vi "testserverstream.vi"() -> ()   [LabVIEW 2016]
uses:
  tls classes/connection creator/server acceptor/server acceptor.lvclass
  C:/Users/IEUser/Desktop/libasynclvtls/tls classes/connection creator/connection creator.lvclass
  tls classes/engine context/engine context.lvclass
  tls classes/connection/connection.lvclass
  tls classes/connection creator/connection creator.lvclass
panel:
  out "error out 2":errorcluster
  out "error out":errorcluster
  out "output cluster":cluster{"error code":i32, "data":string}
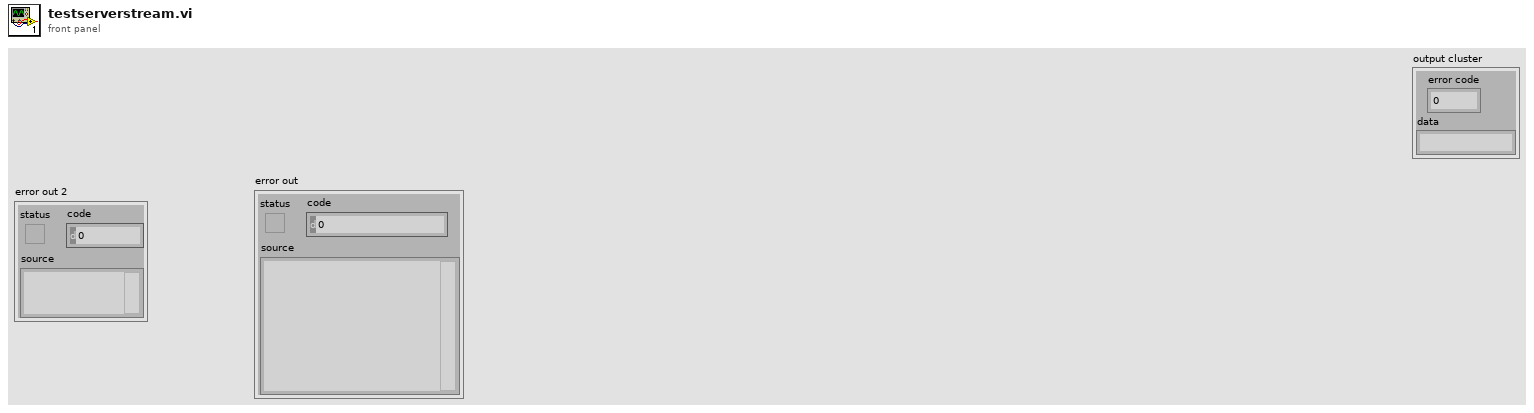
[diagram p1: front panel]
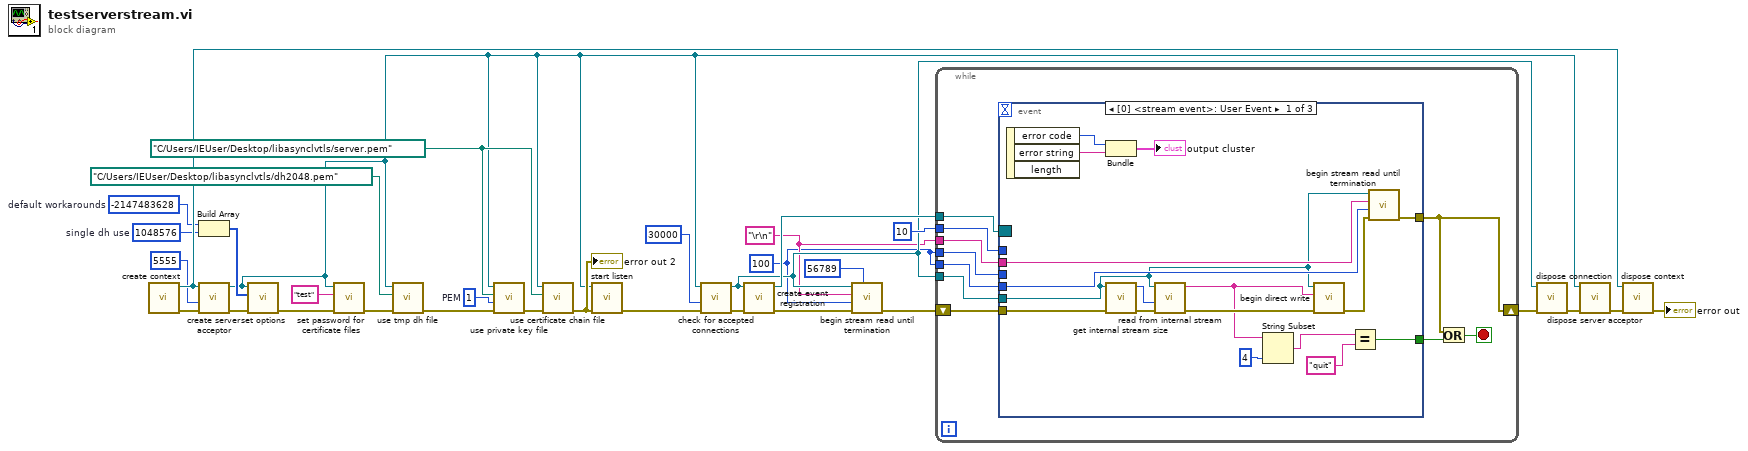
[diagram p0: block diagram]
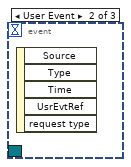
[diagram p2: hidden frame]
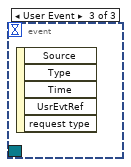
[diagram p3: hidden frame]
diagram:
  w4 = 1  # PEM
  w7 = "\r\n" ("termination")
  w17 = path "C:/Users/IEUser/Desktop/libasynclvtls/server.pem" ("cert chain file")
  w20 = -2147483628  # default workarounds
  w21 = 1048576  # single dh use
  w6 = 100 ("bytes to read")
  n1 = call "create context.vi"() -> ("error out"=w24:errorcluster, "engine context out"=w23:refnum<class "engine context.lvclass">)  [unwired: 10 in]
  n2 = Build Array(w20, w21) -> (w9:i32[])
  n3 = call "create server acceptor.vi"("error in"=w24, "port"=u16 5555, "engine context in"=w23) -> ("error out"=w22:errorcluster, "server acceptor out"=w8:refnum<class "server acceptor.lvclass">)  [unwired: 7 in]
  n4 = call "set options.vi"("error in"=w22, "options"=w9, "connection creator in"=w8) -> ("error out"=w19:errorcluster)  [unwired: 8 in]
  n5 = call "set password for certificate files.vi"("error in"=w19, "password"="test" ("file"), "connection creator in"=w8) -> ("error out"=w3:errorcluster)  [unwired: 8 in]
  n6 = call "use tmp dh file.vi"("error in"=w3, "tmp dh file"=path "C:/Users/IEUser/Desktop/libasynclvtls/dh2048.pem", "connection creator in"=w8) -> ("error out"=w2:errorcluster)  [unwired: 8 in]
  n7 = call "use private key file.vi"("error in"=w2, "format"=w4, "private key file"=w17, "connection creator in"=w8) -> ("error out"=w1:errorcluster)  [unwired: 7 in]
  n8 = call "use certificate chain file.vi"("error in"=w1, "cert chain file"=w17, "connection creator in"=w8) -> ("error out"=w16:errorcluster)  [unwired: 8 in]
  "error out 2" <- w16
  n9 = call "start listen.vi"("error in"=w16, "server acceptor in"=w8) -> ("error out"=w15:errorcluster)  [unwired: 9 in]
  n10 = call "check for accepted connections.vi"("error in"=w15, "timeout"=30000, "server acceptor in"=w8) -> ("error out"=w14:errorcluster, "connection"=w11:refnum<class "connection.lvclass">)  [unwired: 7 in]
  n11 = call "create event registration.vi"("error in"=w14, "connection in"=w11) -> ("error out"=w31:errorcluster, "Event Registration Refnum"=w32:refnum<event-registration>)  [unwired: 8 in]
  n12 = call "begin stream read until termination.vi"("id"=u32 56789, "error in"=w31, "max bytes to read"=w6, "termination"=w7, "connection in"=w11) -> ("error out"=w29:errorcluster)  [unwired: 6 in]
  n13 = while {
    tunnel: w32 -> [w42]
    shift-right: [w36] -> w26
    shift-left: w29 -> [w41]
    tunnel: w11 -> [w40]
    tunnel: 10 ("bytes to read") -> [w39]
    tunnel: w6 -> [w38]
    tunnel: w7 -> [w34]
    tunnel: w6 -> [w33]
    stop <- w37 stop-if-true
    n14 = event shown="[0] <stream event>: User Event" {
      selector: w42 -> [_ _ _]
      dyn-events: _ -> [_ _ _]
      timeout: _ -> [_ _ _]
      tunnel: w41 -> [w46 _ _]
      tunnel: w40 -> [w47 _ _]
      tunnel: [w53 _ _] -> w36
      tunnel: w39 -> [_ _ _]
      tunnel: w38 -> [_ _ _]
      tunnel: [w56 _ _] -> w35
      tunnel: w34 -> [w52 _ _]
      tunnel: w33 -> [w51 _ _]
      event User Event {
        n15 = event-data() -> ("error code"=w59:i32, "error string"=w55:string)  [unwired: 1 in, 1 out]
        n16 = Bundle("error code"=w59, "error string"=w55) -> (→"output cluster":cluster{"error code":i32, "error string":string})  [unwired: 1 in]
        n17 = call "get internal stream size.vi"("error in"=w46, "connection in"=w47) -> ("error out"=w49:errorcluster, "size"=w50:u64)  [unwired: 8 in]
        n18 = call "read from internal stream.vi"("error in"=w49, "max length"=w50, "connection in"=w47) -> ("error out"=w48:errorcluster, "buffer"=w44:string)  [unwired: 7 in]
        n19 = String Subset(string=w44, length (rest)=4 ("length (rest)")) -> (substring=w43:string)  [unwired: 1 in]
        n20 = call "begin direct write.vi"("error in"=w48, "data"=w44, "connection in"=w47) -> ("error out"=w54:errorcluster)  [unwired: 8 in]
        n21 = Equal?(x=w43, y="quit") -> (x = y?=w56:bool)
        n22 = call "begin stream read until termination.vi"("error in"=w54, "max bytes to read"=w51, "termination"=w52, "connection in"=w47) -> ("error out"=w53:errorcluster)  [unwired: 7 in]
      }
      event User Event {
        n23 = event-data() -> ()  [unwired: 1 in, 5 out]
      }
      event User Event {
        n24 = event-data() -> ()  [unwired: 1 in, 5 out]
      }
    }
    n25 = Or(x=w36, y=w35) -> (x .or. y?=w37:bool)
  }
  n26 = call "dispose connection.vi"("error in"=w26, "connection in"=w11) -> ("error out"=w28:errorcluster)  [unwired: 9 in]
  n27 = call "dispose server acceptor.vi"("error in"=w28, "server acceptor in"=w8) -> ("error out"=w27:errorcluster)  [unwired: 9 in]
  n28 = call "dispose context.vi"("error in"=w27, "engine context out"=w23) -> ("error out"=→"error out":errorcluster)  [unwired: 9 in]
